vi "Set Save Settings.vi"(7 "Remove block diagram (false)":bool, 8 "error in (no error)":errorcluster, 9 "Remove front panel (false)":bool, 10 "ProjectItem Refnum":refnum<vi>, 11 "SDIST in":refnum<class "NI_AB_API_DSDIST.lvclass">) -> (0 "error out":errorcluster, 3 "SDIST out":refnum<class "NI_AB_API_DSDIST.lvclass">)   [LabVIEW 2020, in "NI_AB_API_DSDIST.lvclass"]
uses:
  <vilib>/AppBuilder/AB_API/DSDIST/NI_AB_API_DSDIST.lvclass
  <vilib>/AppBuilder/AB_API/SDIST/NI_AB_API_SDIST.lvclass
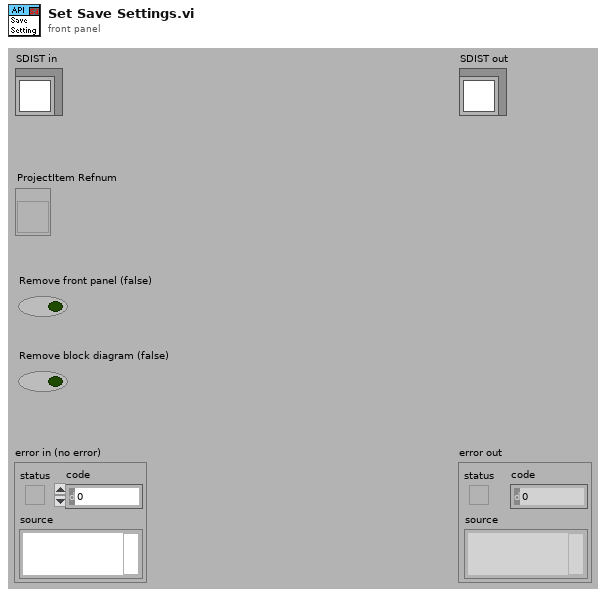
[diagram p1: front panel]
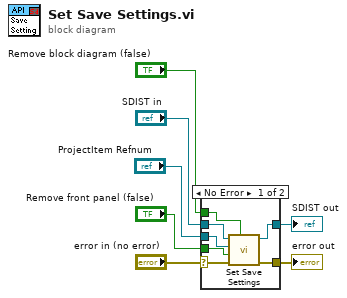
[diagram p0: block diagram]
diagram:
  n1 = case shown="No Error" "error in (no error)" {
    selector: "error in (no error)" -> [w12 w16]
    tunnel: [w11 w16] -> w6
    tunnel: [w13 w15] -> w4
    tunnel: "SDIST in" -> [w14 w15]
    tunnel: "ProjectItem Refnum" -> [w10 _]
    tunnel: "Remove block diagram (false)" -> [w9 _]
    tunnel: "Remove front panel (false)" -> [w8 _]
    frame No Error {
      n2 = call-parent "Set Save Settings.vi"("Remove block diagram (false)"=w9, "error in (no error)"=w12, "Remove front panel (false)"=w8, "ProjectItem Refnum"=w10, "SDIST in"=w14) -> ("error out"=w11:errorcluster, "SDIST out"=w13:refnum<class "NI_AB_API_DSDIST.lvclass">)  [unwired: 5 in]
    }
    frame Error {
    }
  }
  "error out" <- w6
  "SDIST out" <- w4
